vi "MDOAcquire Data from Hardware.vi"(7 "error in (no error)":errorcluster, 10 "Hardware Configuration":T1 {"SyncMode" items=["INTERNAL"=0, "EXTERNAL_MASTER"=1, "DI_SYN1_RISE"=2, "DI_SYN1_FALL"=3, "DI_SYN2_RISE"=6, "DI_SYN2_FALL"=7]}) -> (0 "error out":errorcluster, 2 "Current":dbl[](array[numeric]), 3 "Voltage":dbl[](array[numeric]))   [LabVIEW 2020]
doc: "Generates sample waveforms according to the signal type in the HW Config input."
uses:
  controls/MDOHW Configuration.ctl
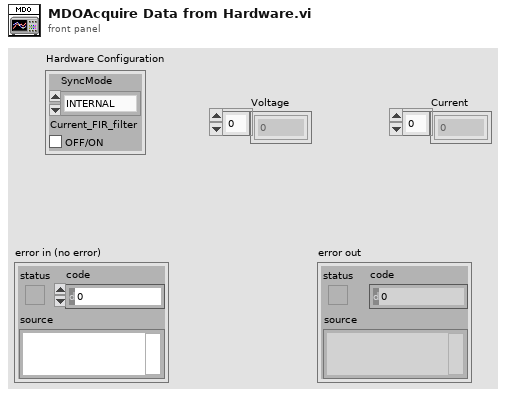
[diagram p1: front panel]
types:
  T1 = typedef "MDOHW Configuration.ctl" = cluster{"SyncMode":u32, "Current_FIR_filter":bool}
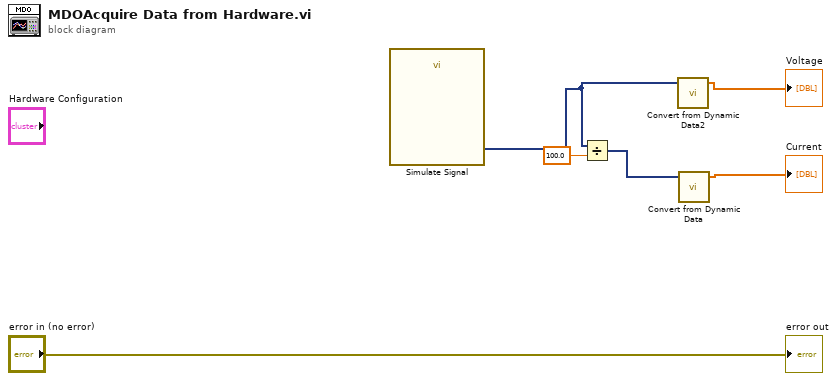
[diagram p0: block diagram]
diagram:
  n1 = call "Simulate Signal"() -> ("Sine with Uniform Noise"=w2:dynamicdata)  [unwired: 14 in, 1 out]
  n2 = Divide(x=w2, y=100.0) -> (x/y=w4:dynamicdata)
  n3 = call "Convert from Dynamic Data2"("Dynamic Data Type"=w2) -> ("Array"=→"Voltage":dbl[])  [unwired: 3 in]
  n4 = call "Convert from Dynamic Data"("Dynamic Data Type"=w4) -> ("Array"=→"Current":dbl[])  [unwired: 3 in]
  "error out" <- "error in (no error)"
